vi "ir.vi"(11 "Port":u8) -> (3 "Direction":i16)   [LabVIEW 2010, in "LASA Beta.lvrbt"]
doc: "Receives the information from a HiTechnic IR Sensor. The output contains a direction 0-9 (0 = no signal; 1=left of sensor; 9=right of sensor; 5=dead-on sensor)."
uses:
  LASA Beta.lvrbt
  <vilib>/NXT/HiTechnic/HiTechnic Controls/HiTechnic Port.ctl
  <vilib>/NXT/Block Support/NXT_InputPort.ctl
  <vilib>/NXT/HiTechnic/HiTechnic Read/HiTechnic IRSeeker Sensor_AC all.vi
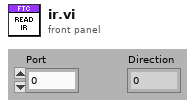
[diagram p1: front panel]
types:
  T1 = typedef "HiTechnic Port.ctl" = cluster{"Port":T2, "MUX Port":u8}
  T2 = typedef "NXT_InputPort.ctl" = u8
  T3 = cluster{"Direction (0-9)":i16, "Signal Strength (Array)":u8[]}
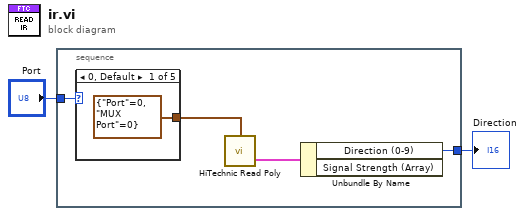
[diagram p0: block diagram]
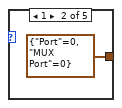
[diagram p2: hidden frame]
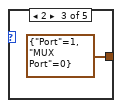
[diagram p3: hidden frame]
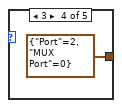
[diagram p4: hidden frame]
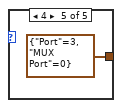
[diagram p5: hidden frame]
diagram:
  n1 = stacked-sequence {
    tunnel: "Port" -> [w6]
    tunnel: [w3] -> w1
    frame #0 {
      n2 = case shown="0, Default" w6 {
        tunnel: [T1 {"Port"=0, "MUX Port"=0} ("Port/MUX") T1 {"Port"=0, "MUX Port"=0} ("Port/MUX") T1 {"Port"=1, "MUX Port"=0} ("Port/MUX") T1 {"Port"=2, "MUX Port"=0} ("Port/MUX") T1 {"Port"=3, "MUX Port"=0} ("Port/MUX")] -> w5
        frame 0, Default {
        }
        frame 1 {
        }
        frame 2 {
        }
        frame 3 {
        }
        frame 4 {
        }
      }
      n3 = call-poly <vilib>:"HiTechnic Read Poly.vi"("Port/MUX"=w5) -> ("All Info"=w4:T3)  [unwired: 2 in, 1 out]
      n4 = Unbundle By Name(w4) -> ("Direction (0-9)"=w3:i16)  [unwired: 1 out]
    }
  }
  "Direction" <- w1
